vi "Start.vi"(8 "error in (no error)":errorcluster, 11 "ISeries Actor in":refnum<class "ISeries Actor.lvclass">) -> (0 "error out":errorcluster, 3 "ISeries Actor out":refnum<class "ISeries Actor.lvclass">)   [LabVIEW 2023, in "ISeries Actor.lvlib" / "ISeries Actor.lvclass"]
uses:
  ISeries Actor.lvclass
  <vilib>/ErrorRing/Error Ring.xnode
  <vilib>/Utility/error.llb/Error Cluster From Error Code.vi
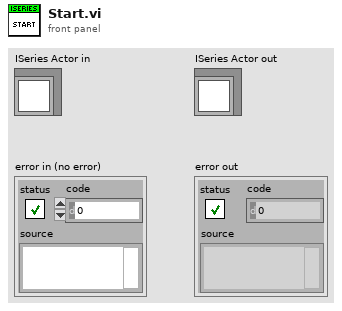
[diagram p1: front panel]
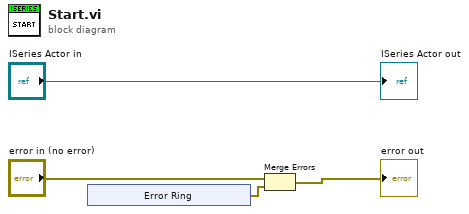
[diagram p0: block diagram]
diagram:
  n1 = xnode "Error Ring"() -> ("error out"=w1:errorcluster)
  n2 = Merge Errors("error in (no error)", w1) -> (→"error out":errorcluster)
  "ISeries Actor out" <- "ISeries Actor in"
